vi "FPGA.vi"() -> ()   [LabVIEW 2015]
uses:
  LCD Command.ctl
  <vilib>/rvi/Emulation/niFpgaGetClockAttributes.vi
  <vilib>/rvi/Emulation/niFpgaSctlEmulationGetInTimedLoop.vi
  <vilib>/rvi/Emulation/niFpgaEmulationReportErrorSimple.vi
  <vilib>/EmbeddedDisplay/Hitachi HD44780/FPGA/Internal/LCD Command.vi
  <vilib>/EmbeddedDisplay/Hitachi HD44780/FPGA/Public/Command Handler (8 Bits).vi
  <vilib>/rvi/Emulation/niFpgaProcessEmulError.vi
  <vilib>/rvi/Emulation/niFpgaCriticalErrorInLSC.vi
  <vilib>/rvi/eio/common/nirviEmuTemplateMethod_errors.vi
  <vilib>/rvi/interface/RandomDataEmulation/niFpgaRandomDataHandleErrors.vi
  <vilib>/eio/EIONode/EIONode.xnode
  <vilib>/rvi/DataTransferAndStorage/Container/XNode/niFpgaContainer.xnode
  <vilib>/rvi/interface/RandomDataEmulation/nirviRandomDataFpgaReadWriteTemplate.vi
  <vilib>/EmbeddedDisplay/Hitachi HD44780/FPGA/HD44780 FPGA.lvlib
panel:
  out "POT":fxp<+/-,24,5>
  out "Temp Senesor":fxp<+/-,24,5>
  in  "LCD Command":T1={"device index (-1)"=-1, "operation (0)"=0}
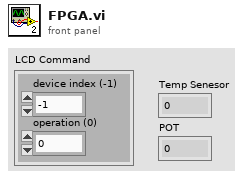
[diagram p1: front panel]
types:
  T1 = typedef "LCD Command.ctl" = cluster{"device index (-1)":i8, "operation (0)":u32}
  T2 = cluster{"RS":refnum<k21>, "R/W":refnum<k21>, "E1":refnum<k21>, "E2":refnum<k21>, "DB0":refnum<k21>, "DB1":refnum<k21>, "DB2":refnum<k21>, "DB3":refnum<k21>, "DB4":refnum<k21>, "DB5":refnum<k21>, "DB6":refnum<k21>, "DB7":refnum<k21>}
  T3 = cluster{"device index (-1)":i8, "operation (0)":u32}
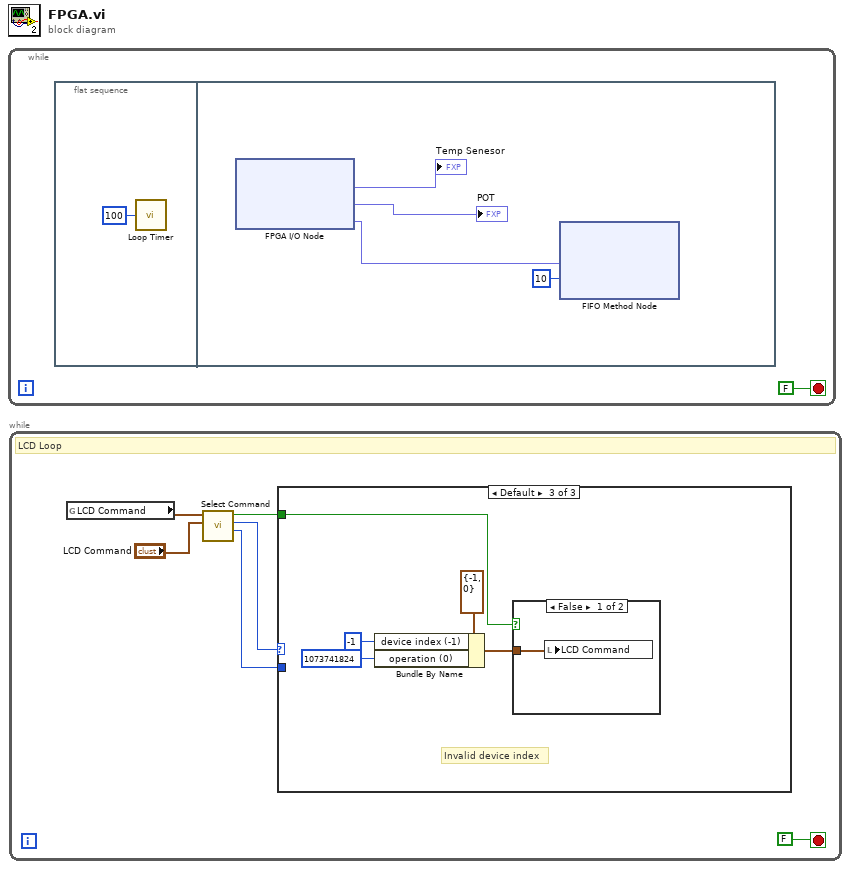
[diagram p0: block diagram]
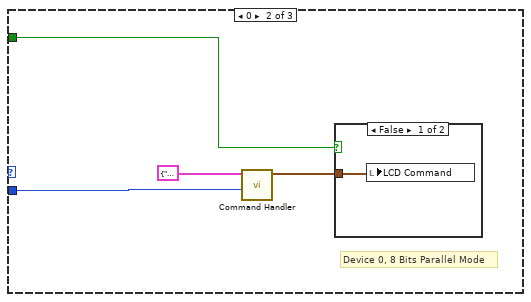
[diagram p3: hidden frame]
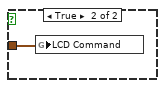
[diagram p4: hidden frame]
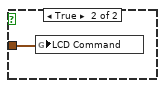
[diagram p5: hidden frame]
diagram:
  n1 = while {
    stop <- FALSE stop-if-true
    n2 = flat-sequence {
      frame #0 {
        n3 = call "Loop Timer"("Count(uSec)"=u32 100) -> ()  [unwired: 1 out]
      }
      frame #1 {
        n4 = xnode "FPGA I/O Node"() -> ("Temp Senesor"=→"Temp Senesor":fxp<+/-,24,5>, "POT"=→"POT":fxp<+/-,24,5>, "Signal"=w4:fxp<+/-,24,5>)  [unwired: 3 in, 3 out]
        n5 = xnode ("FIFO Method Node")("Element"=w4, "Timeout"=10) -> ()  [unwired: 1 in, 2 out]
      }
    }
  }
  n6 = while {
    stop <- FALSE stop-if-true
    # "LCD Loop"
    n7 = global read "LCD Command.vi" "LCD Command"() -> (w7:T3)
    n8 = call <vilib>:"Select Command.vi"("Host LCD Command"="LCD Command", "FPGA LCD Command"=w7) -> ("operation"=w9:u32, "device index"=w10:i8, "FPGA? True : False"=w8:bool)  [unwired: 7 in]
    n9 = case shown="Default" w10 {
      tunnel: w9 -> [_ w16 _]
      tunnel: w8 -> [_ w15 w23]
      frame -1 {
        # "IDLE State"
      }
      frame 0 {
        # "Device 0, 8 Bits Parallel Mode"
        n10 = call-poly <vilib>:"Command Handler.vi"("operation"=w16, "device connection map in"=T2 {"RS"="LCD Reg SEL", "R/W"="LCD R/W", "E1"="LCD EN", "E2"="LCD EN", "DB0"="LCD Data 0", "DB1"="LCD Data 1", "DB2"="LCD Data 2", "DB3"="LCD Data 3", "DB4"="LCD Data 4", "DB5"="LCD Data 5", "DB6"="LCD Data 6", "DB7"="LCD Data 7"}) -> ("result"=w14:T3)  [unwired: 9 in]
        n11 = case shown="False" w15 {
          tunnel: w14 -> [w17 w18]
          frame False {
            n12 = local write "LCD Command"(w17) -> ()
          }
          frame True {
            n13 = global write "LCD Command.vi" "LCD Command"(w18) -> ()
          }
        }
      }
      frame Default {
        # "Invalid device index"
        n14 = Bundle By Name(cluster=T3 {"device index (-1)"=-1, "operation (0)"=0} ("LCD Command"), "device index (-1)"=i8 -1 ("LCD_device index (-1)"), "operation (0)"=u32 1073741824 ("LCD_operation (0)")) -> (w19:T3)
        n15 = case shown="False" w23 {
          tunnel: w19 -> [w24 w25]
          frame False {
            n16 = local write "LCD Command"(w24) -> ()
          }
          frame True {
            n17 = global write "LCD Command.vi" "LCD Command"(w25) -> ()
          }
        }
      }
    }
  }
